vi "Nums2Str.vi"(7 "Values":dbl[](array[numeric])) -> (8 "Array":string[](array[string]))   [LabVIEW 2024]
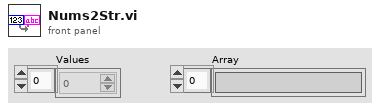
[diagram p1: front panel]
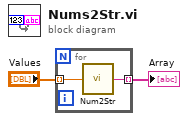
[diagram p0: block diagram]
diagram:
  n1 = for {
    tunnel: "Values" -> [w4] mode=indexing
    tunnel: [w3] -> w1 mode=indexing
    n2 = call "Num2Str.vi"("value"=w4) -> ("output string"=w3:string)  [unwired: 14 in]
  }
  "Array" <- w1
